vi "Has Tag.vi"(8 "error in (no error)":errorcluster, 10 "Tag":string, 11 "FeedItem in":refnum<class "FeedItem.lvclass">) -> (0 "error out":errorcluster, 2 "Boolean":bool, 3 "FeedItem out":refnum<class "FeedItem.lvclass">)   [LabVIEW 2020, in "FeedItem.lvclass"]
uses:
  <vilib>/NI_RSS/FeedItem/FeedItem.lvclass
  <vilib>/NI_RSS/FeedItem/FeedItem.lvclass/FeedItem.ctl
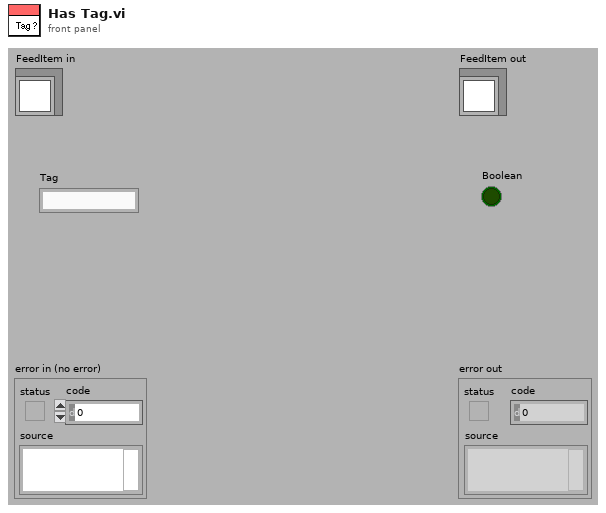
[diagram p1: front panel]
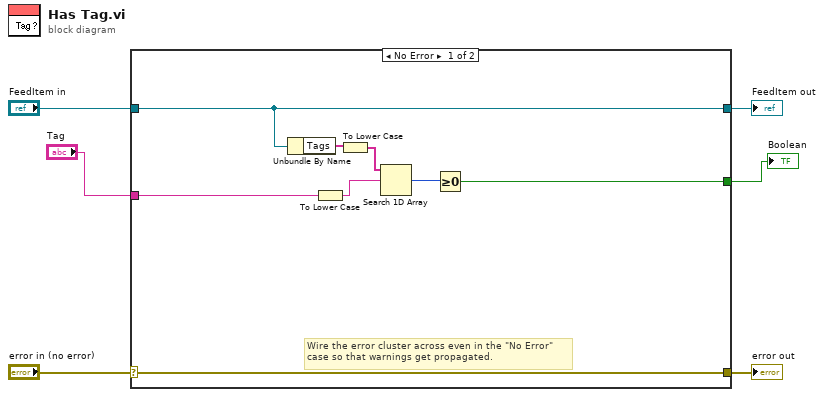
[diagram p0: block diagram]
diagram:
  n1 = case shown="No Error" "error in (no error)" {
    selector: "error in (no error)" -> [w14 w16]
    tunnel: [w14 w16] -> w5
    tunnel: [w13 w15] -> w3
    tunnel: "FeedItem in" -> [w13 w15]
    tunnel: "Tag" -> [w9 _]
    tunnel: [w7 _] -> w1
    frame No Error {
      # "Wire the error cluster across even in the \"No Error\"\ncase so that warnings get propagated."
      n2 = Unbundle By Name(w13) -> ("Tags"=w12:string[])
      n3 = To Lower Case(string=w9) -> (all lower case string=w10:string)
      n4 = To Lower Case(string=w12) -> (all lower case string=w11:string[])
      n5 = Search 1D Array(1D array=w11, element=w10) -> (index of element=w8:i32)  [unwired: 1 out]
      n6 = Greater Or Equal To 0?(x=w8) -> (x >= 0?=w7:bool)
    }
    frame Error {
    }
  }
  "error out" <- w5
  "FeedItem out" <- w3
  "Boolean" <- w1
